vi "getEventSettingVersions.vi"(11 "UserEvents in":refnum<class "UserEvents.lvclass">) -> (2 "EventSettingVersions":refnum<user-event>, 3 "UserEvents out":refnum<class "UserEvents.lvclass">)   [LabVIEW 2016, in "UserEvents.lvclass"]
uses:
  UserEvents.lvclass
  DataTypes/Topics/EventSettingVersions.ctl
  DataTypes/Topics/Parts/Timestamp.ctl
  UserEvents.lvclass/UserEvents.ctl
  DataTypes/Topics/M1M3SupportTopics.lvlib
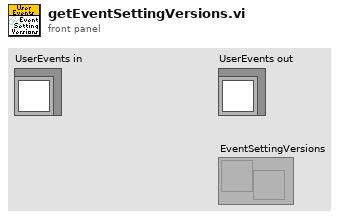
[diagram p1: front panel]
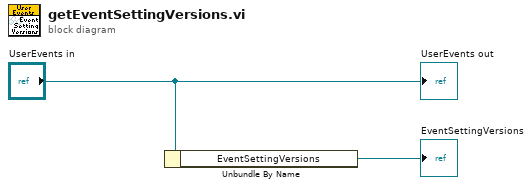
[diagram p0: block diagram]
diagram:
  n1 = Unbundle By Name("UserEvents in") -> ("EventSettingVersions"=→"EventSettingVersions":refnum<user-event>)
  "UserEvents out" <- "UserEvents in"
